vi "Send New Message.vi"(6 "Receiving Actor":refnum<class "Message Enqueuer.lvclass">, 7 "Priority":T1 caption="Message Priority (Normal)", 8 "error in (no error)":errorcluster, 9 "Message":refnum<class "Message.lvclass">, 10 "Time Stamp":timestamp, 11 "Message Enqueuer in":refnum<class "Message Enqueuer.lvclass">) -> (0 "error out":errorcluster, 3 "Message Enqueuer out":refnum<class "Message Enqueuer.lvclass">)   [LabVIEW 2023, in "Monitored Actor.lvlib" / "New Message Msg.lvclass"]
doc: "Sends the <b>New Message Msg.lvclass</b> message.\n\nThis message will call <b>New Message.vi</b> on the <b>Monitored Actor.lvlib:Classic Logger.lvclass</b> actor.\n\n<b>New Message.vi Description</b>\nCalled any time a monitored actor receives a message\n\nCopyright: MGI 2016\nAuthor: Derek Trepanier"
uses:
  New Message Msg.lvclass
  builds/Engine/Actor Framework.lvlibp/1abvi3w/vi.lib/ActorFramework/Message Enqueuer/Message Enqueuer.lvclass
  builds/Engine/Actor Framework.lvlibp/1abvi3w/vi.lib/ActorFramework/Message Enqueuer/Message Priority.ctl
  builds/Engine/Actor Framework.lvlibp/1abvi3w/vi.lib/ActorFramework/Message/Message.lvclass
  New Message Msg.lvclass/New Message Msg.ctl
  C:/Users/Public/Documents/Development/builds/Engine/Actor Framework.lvlibp/1abvi3w/vi.lib/ActorFramework/Message/Message.lvclass
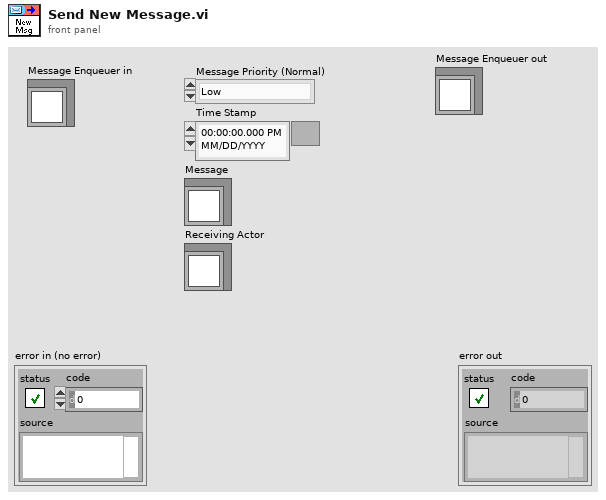
[diagram p1: front panel]
types:
  T1 = typedef "Actor Framework.lvlibp/Message Enqueuer.lvclass/Message Priority.ctl" = enum16{"Low", "Normal", "High"}
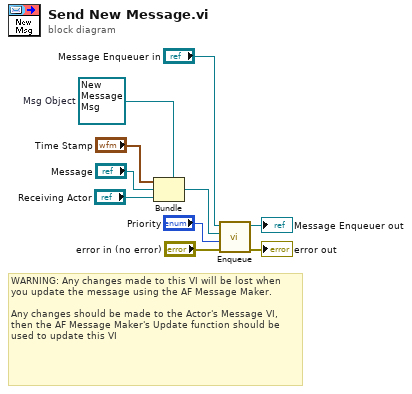
[diagram p0: block diagram]
diagram:
  w7 = refnum<class "New Message Msg.lvclass"> refnum  # Msg Object
  # "WARNING: Any changes made to this VI will be lost when you update the message using the AF Message Maker.\n\nAny changes should be made to the Actor's Message VI, then the AF Message Maker's Update function should be used to update this VI"
  n1 = Bundle(cluster=w7, "Time Stamp", "Message", "Receiving Actor") -> (w2:refnum<class "New Message Msg.lvclass">)
  n2 = call "Enqueue.vi"("error in (no error)"="error in (no error)", "Message Priority (Normal)"="Priority", "Message"=w2, "Message Enqueuer in"="Message Enqueuer in") -> ("error out"=→"error out":errorcluster, "Message Enqueuer out"=→"Message Enqueuer out":refnum<class "Message Enqueuer.lvclass">)  [unwired: 6 in]
